vi "ATF Storage-RT_Main.vi"   [LabVIEW 2022 SP3]
uses:
  RT Controls/ATF Storage-RT main.ctl
  RT Support/ATF Storage-RT_Global_R.vi
panel:
  # "RT main ATF-Storage"
types:
  T1 = typedef "ATF Storage-RT main.ctl" = enum16{"initialise", "Wait for connection", "Wait for command"}
  T2 = enum16{"Init", "Read 'All'", "Read 'n'", "Read '1'", "Write '1'", "Write 'n'", "Write 'All'"}
  T3 = cluster{"Drive Control":cluster{"En_Drive_A":bool, "En_Drive_L":bool, "Exit_Drive_A":bool, "Exit_Drive_L":bool}, "Drive_ATF Control":cluster{"S.Freq":dbl, "Ramp up Time":dbl, "Ramp down Time":dbl, "Drive Speed":dbl, "Drive condition":dbl}, "Drive_LOX Control":cluster{"S.Freq":dbl, "Ramp up Time":dbl, "Ramp down Time":dbl, "Drive Speed":dbl, "Drive condition":dbl}, "Aconnection ID":refnum<k5>, "Lconnection ID":refnum<k5>, "Loop Control":cluster{"Start DAQ":bool, "Stop DAQ":bool, "RT Stop":bool, "RT Exit":bool, "Start Seq":bool}}
  T4 = typedef "ATF Storage-Data FIFO.ctl" = cluster{"RD":cluster{"AI_V_Data RD":refnum<queue>, "AI_C_Data RD":refnum<queue>, "AO_Data RD":refnum<queue>, "DI_Data RD":refnum<queue>, "ACC_Data RD":refnum<queue>, "TC_Data RD":refnum<queue>, "Drive_A_C RD":refnum<queue>, "Drive_A_D RD":refnum<queue>, "Drive_L_C RD":refnum<queue>, "Drive_L_D RD":refnum<queue>, "DI Data":refnum<queue>, "DO_Data RD":refnum<queue>}, "ERR":refnum<queue>}
  T5 = cluster{"Channel List":cluster{"AI Channel list":tag[], "AO Channel list":tag[], "DO Channel list ":tag[], "DI Channel list":tag[]}, "Device List":cluster{"AO Cards":tag[], "AI Cards":tag[], "DI Cards":tag[], "DO Cards":tag[]}}
  T6 = cluster{"AO config":cluster{"Channel_Name":string, "Channel_Number":string, "Default_Value":dbl, "Units":string}[], "AI config":cluster{"Channel_Name":string, "Channel_Number":string, "Pre_Scale_min":dbl, "Pre_Scale_max":dbl, "Sensor_min":dbl, "Sensor_max":dbl, "Units":string}[], "DI config":cluster{"Channel_Name":string, "Channel_Number":string, "Default_Value":bool, "DI invert?":bool}[], "DO config":cluster{"Channel_Name":string, "Channel_Number":string, "Default_Value":bool, "DO invert?":bool}[], "TC config":cluster{"Channel_Name":string, "Channel_Number":string, "Pre_Scale_min":dbl, "Pre_Scale_max":dbl, "units":i32, " type":i32}[], "ACC config":cluster{"Channel_Name":string, "Channel_Number":string, "Pre_Scale_min":dbl, "Pre_Scale_max":dbl, "Terminal configuration":i32, "Sensitivity":dbl, "Sensitivity units":i32}[], "SG config":cluster{"Channel_Name":string, "Channel_Number":string, "Pre_Scale_min":dbl, "Pre_Scale_max":dbl}[], "Strain Gauge Settings":cluster{"poisson ratio":dbl, "nominal gage resistance":dbl, "gage factor":dbl}, "Bridge Settings":cluster{"voltage excitation value":dbl, "voltage excitation source":i32, "initial bridge voltage":dbl, "lead wire resistance":dbl, "strain configuration":i32}, "Sample Rate":cluster{"AI Sample Rate":dbl[], "AO Sample Rate":dbl[], "DI Sample Rate":dbl[], "TC Sample Rate":dbl[], "DO Sample Rate":dbl[], "SG Sample Rate":dbl[], "ACC Sample Rate":dbl[]}}
  T7 = enum16{"Init", "Read", "Write 'All'", "Write 'n'", "Write Safe Value", "Write Start Time", "Overwrite Pattern", "Overwrite Pattern with Start", "Append Pattern", "Start Pattern Mode", "Abort Pattern Mode", "Read 1"}
  T8 = cluster{"Start DAQ":bool, "Stop DAQ":bool, "RT Stop":bool, "RT Exit":bool, "Start Seq":bool}
  T9 = cluster{"AO Cards":tag[], "AI Cards":tag[], "DI Cards":tag[], "DO Cards":tag[]}
  T10 = cluster{"AI Channel list":tag[], "AO Channel list":tag[], "DO Channel list ":tag[], "DI Channel list":tag[]}
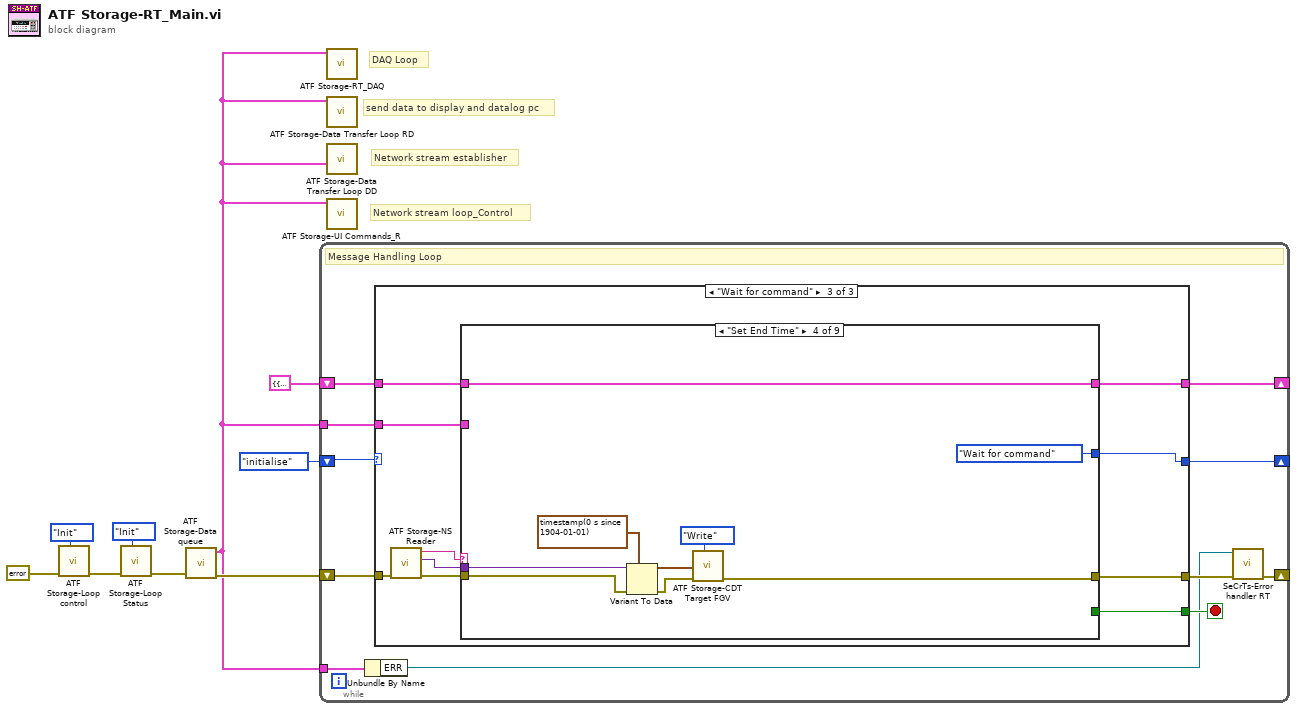
[diagram p0: block diagram]
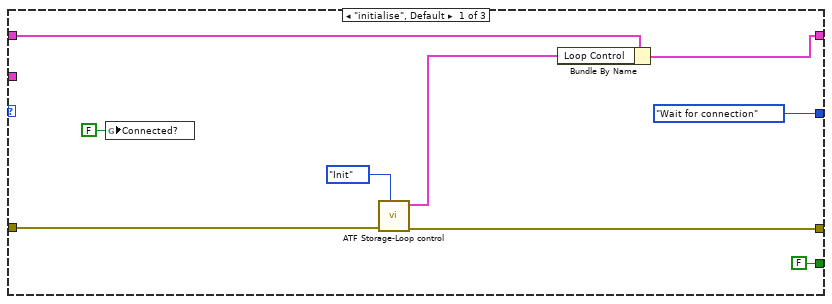
[diagram p2: hidden frame]
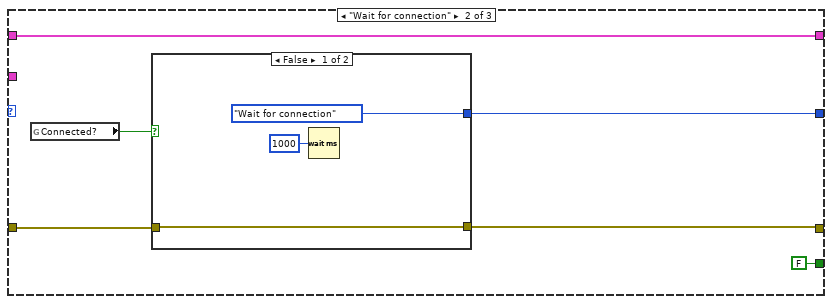
[diagram p3: hidden frame]
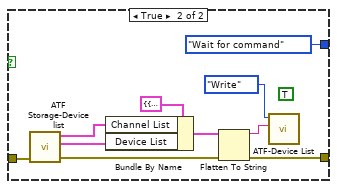
[diagram p4: hidden frame]
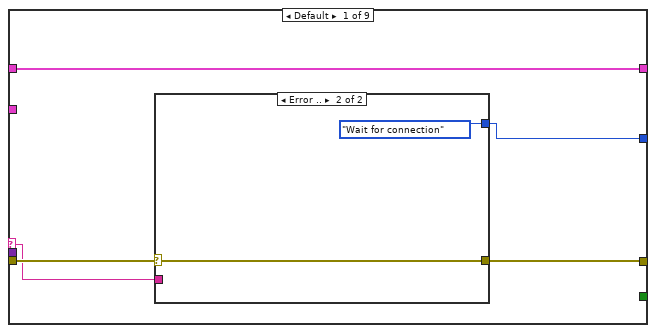
[diagram p5: hidden frame]
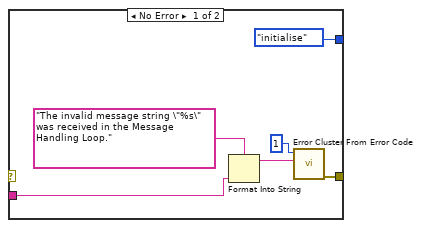
[diagram p6: hidden frame]
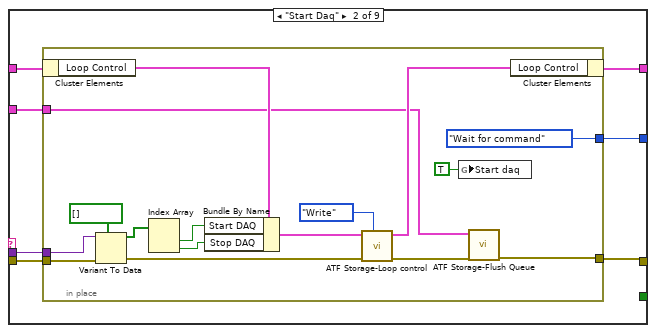
[diagram p7: hidden frame]
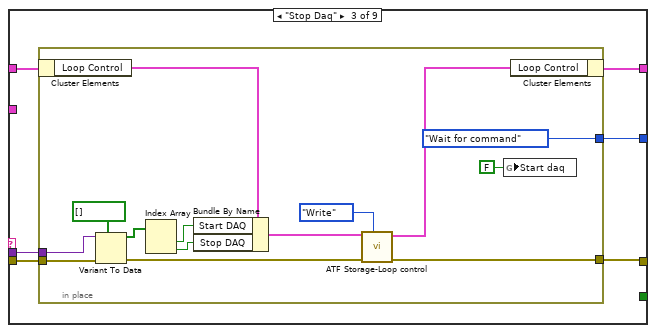
[diagram p8: hidden frame]
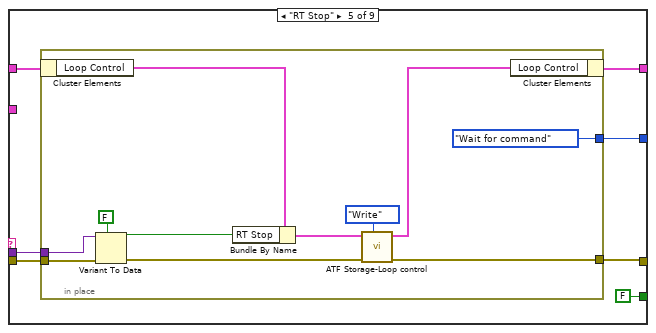
[diagram p9: hidden frame]
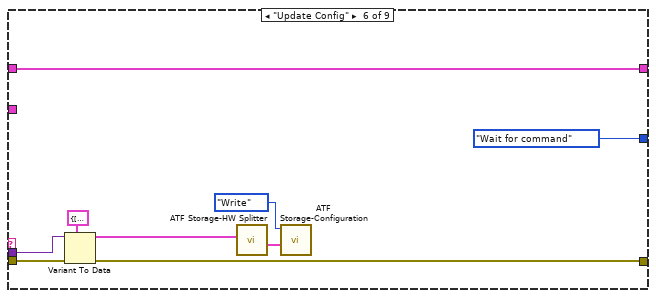
[diagram p10: hidden frame]
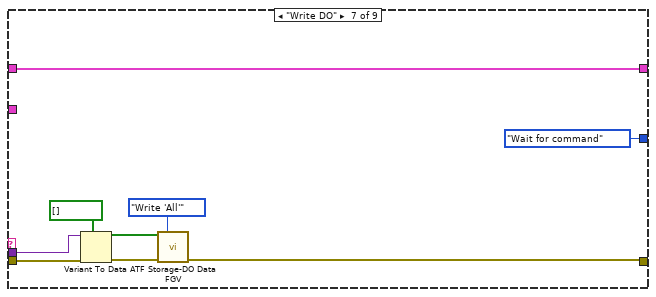
[diagram p11: hidden frame]
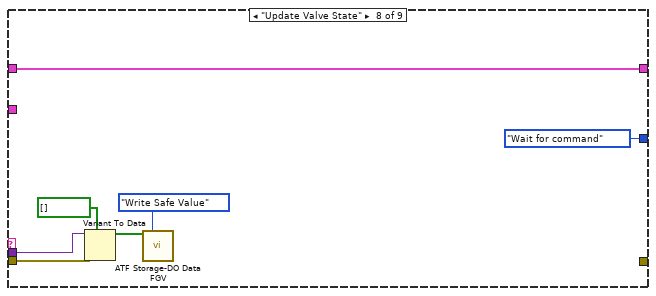
[diagram p12: hidden frame]
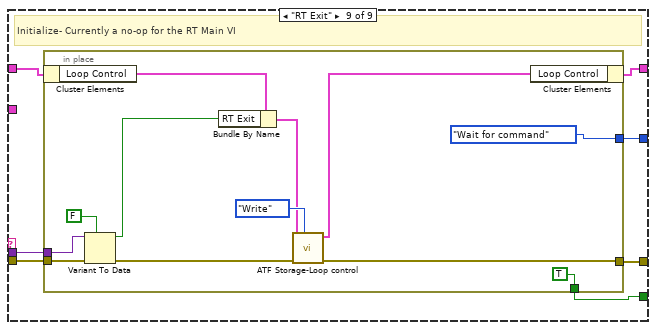
[diagram p13: hidden frame]
diagram:
  # "send data to display and datalog pc"
  # "Network stream establisher"
  # "DAQ Loop"
  # "Network stream loop_Control"
  n1 = call "ATF Storage-Loop control.vi"("Action"=enum16{"Init", "Write", "Read"}."Init", "error in (no error)"=errorcluster {"status"=FALSE, "code"=0, "source"=""} ("error constant")) -> ("error Out"=w3:errorcluster)  [unwired: 8 in, 1 out]
  n2 = call "ATF Storage-Loop Status.vi"("Option"=T2."Init", "error in (no error)"=w3) -> ("error out"=w6:errorcluster)  [unwired: 7 in, 2 out]
  n3 = call "ATF Storage-Data queue.vi"("error in"=w6) -> ("Data FIFO Ref"=w1:T4, "error out"=w8:errorcluster)  [unwired: 8 in]
  n4 = while {
    shift-right: [w15] -> _
    shift-left: w8 -> [w20]
    shift-right: [w17] -> _
    shift-left: T3 {"Drive Control"={"En_Drive_A"=FALSE, "En_Drive_L"=FALSE, "Exit_Drive_A"=FALSE, "Exit_Drive_L"=FALSE}, "Drive_ATF Control"={"S.Freq"=0.0, "Ramp up Time"=0.0, "Ramp down Time"=0.0, "Drive Speed"=0.0, "Drive condition"=0.0}, "Drive_LOX Control"={"S.Freq"=0.0, "Ramp up Time"=0.0, "Ramp down Time"=0.0, "Drive Speed"=0.0, "Drive condition"=0.0}, "Aconnection ID"=refnum, "Lconnection ID"=refnum, "Loop Control"={"Start DAQ"=FALSE, "Stop DAQ"=FALSE, "RT Stop"=FALSE, "RT Exit"=FALSE, "Start Seq"=FALSE}} -> [w18]
    tunnel: w1 -> [w14]
    shift-right: [w12] -> _
    shift-left: ATF_Storage-RT_main."initialise" -> [w13]
    tunnel: w1 -> [w11]
    stop <- w19 stop-if-true
    # "Message Handling Loop"
    n5 = Unbundle By Name(w11) -> ("ERR"=w10:refnum<queue>)
    n6 = case shown="\"Wait for command\"" w13 {
      tunnel: w20 -> [w25 w34 w53]
      tunnel: [FALSE FALSE w58] -> w19
      tunnel: w18 -> [w23 w31 w57]
      tunnel: [w22 w31 w56] -> w17
      tunnel: [w24 w33 w55] -> w16
      tunnel: w14 -> [_ _ w54]
      tunnel: [ATF_Storage-RT_main."Wait for connection" w32 w49] -> w12
      frame "initialise", Default {
        n7 = global write "ATF Storage-RT_Global_R.vi" "Connected?"(FALSE ("Connected?")) -> ()
        n8 = call "ATF Storage-Loop control.vi"("Action"=enum16{"Init", "Write", "Read"}."Init", "error in (no error)"=w25) -> ("error Out"=w24:errorcluster, "Loop Control out"=w21:T8)  [unwired: 8 in]
        n9 = Bundle By Name(cluster=w23, "Loop Control"=w21) -> (w22:T3)
      }
      frame "Wait for connection" {
        n10 = global read "ATF Storage-RT_Global_R.vi" "Connected?"() -> (w35:bool)
        n11 = case shown="False" w35 {
          tunnel: w34 -> [w38 w42]
          tunnel: [w38 w40] -> w33
          tunnel: [ATF_Storage-RT_main."Wait for connection" ATF_Storage-RT_main."Wait for command"] -> w32
          frame False {
            n12 = Wait (ms)(milliseconds to wait=u32 1000) -> ()  [unwired: 1 out]
          }
          frame True {
            (unwired) TRUE ("Connected?")
            n13 = call "ATF Storage-Device list.vi"("error in (no error)"=w42) -> ("error out"=w41:errorcluster, "Device List"=w47:T9, "Channel List"=w48:T10)  [unwired: 8 in]
            n14 = Bundle By Name(cluster=T5 {"Channel List"={"AI Channel list"=[], "AO Channel list"=[], "DO Channel list "=[], "DI Channel list"=[]}, "Device List"={"AO Cards"=[], "AI Cards"=[], "DI Cards"=[], "DO Cards"=[]}}, "Channel List"=w48, "Device List"=w47) -> (w44:T5)
            n15 = Flatten To String(anything=w44, error in (no error)=w41) -> (data string=w43:string, error out=w40:errorcluster)  [unwired: 2 in, 1 out]
            n16 = call "ATF-Device List.vi"("DL"=w43, "Enum"=enum16{"Write", "Read"}."Write") -> ()  [unwired: 8 in, 2 out]
          }
        }
      }
      frame "Wait for command" {
        n17 = call "ATF Storage-NS Reader.vi"("error in (no error)"=w53) -> ("error IO"=w52:errorcluster, "Message Data"=w51:variant, "Message"=w50:string)  [unwired: 8 in]
        n18 = case shown="\"Set End Time\"" w50 {
          selector: w50 -> [w59 _ _ _ _ _ _ _ _]
          tunnel: w51 -> [_ w76 w98 w122 w128 w147 w157 w163 w172]
          tunnel: w52 -> [w60 w78 w100 w121 w130 w148 w158 w165 w173]
          tunnel: [w61 w77 w99 w117 w129 w145 w154 _ w171] -> w55
          tunnel: [_ _ _ _ FALSE _ _ _ w170] -> w58
          tunnel: w57 -> [w63 w75 w97 w123 w127 w150 w159 w166 w169]
          tunnel: [w63 w74 w96 w123 w126 w150 w159 w166 w168] -> w56
          tunnel: w54 -> [_ w73 _ _ _ _ _ _ _]
          tunnel: [w62 w72 w95 ATF_Storage-RT_main."Wait for command" w124 ATF_Storage-RT_main."Wait for command" ATF_Storage-RT_main."Wait for command" ATF_Storage-RT_main."Wait for command" w167] -> w49
          frame Default {
            n19 = case shown="Error .." w60 {
              selector: w60 -> [_ w71]
              tunnel: w59 -> [w66 _]
              tunnel: [w65 w71] -> w61
              tunnel: [ATF_Storage-RT_main."initialise" ATF_Storage-RT_main."Wait for connection"] -> w62
              frame No Error {
                n20 = Format Into String(format string="The invalid message string \"%s\" was received in the Message Handling Loop." ("Unknown Message Error Text"), w66) -> (resulting string=w67:string)  [unwired: 2 in, 1 out]
                n21 = call <vilib>:"Error Cluster From Error Code.vi"("error message (\"\")"=w67, "error code (0)"=1) -> ("error out"=w65:errorcluster)  [unwired: 7 in]
              }
              frame Error {
              }
            }
          }
          frame "Start Daq" {
            n22 = in-place {
              in-place-border: w78 -> [w93]
              in-place-border: [w82] -> w77
              in-place-border: w76 -> [w90]
              in-place-border: w73 -> [w81]
              in-place-border: [ATF_Storage-RT_main."Wait for command"] -> w72
              n23 = in-place-cluster #1(w75) -> ("Loop Control"=w89:T8)
              n24 = Variant To Data(error in=w93, type=bool[] [], Variant=w90) -> (data=w86:bool[], error out=w91:errorcluster)
              n25 = Index Array(array=w86) -> (element #1=w85:bool, element #2=w84:bool)  [unwired: 2 in]
              n26 = Bundle By Name(cluster=w89, "Start DAQ"=w85, "Stop DAQ"=w84) -> (w88:T8)
              n27 = call "ATF Storage-Loop control.vi"("Action"=enum16{"Init", "Write", "Read"}."Write", "error in (no error)"=w91, "Loop Control In"=w88) -> ("error Out"=w83:errorcluster, "Loop Control out"=w87:T8)  [unwired: 7 in]
              n28 = global write "ATF Storage-RT_Global_R.vi" "Start daq"(TRUE ("Start daq")) -> ()
              n29 = call "ATF Storage-Flush Queue.vi"("error in (no error)"=w83, "Data FIFO Ref"=w81) -> ("error out"=w82:errorcluster)  [unwired: 9 in]
              n30 = in-place-cluster #1("Loop Control"=w87) -> (w74:T3)
            }
          }
          frame "Stop Daq" {
            n31 = in-place {
              in-place-border: w100 -> [w113]
              in-place-border: [w110] -> w99
              in-place-border: w98 -> [w109]
              in-place-border: [ATF_Storage-RT_main."Wait for command"] -> w95
              n32 = in-place-cluster #2(w97) -> ("Loop Control"=w108:T8)
              n33 = Variant To Data(error in=w113, type=bool[] [], Variant=w109) -> (data=w105:bool[], error out=w111:errorcluster)
              n34 = Index Array(array=w105) -> (element #1=w104:bool, element #2=w103:bool)  [unwired: 2 in]
              n35 = Bundle By Name(cluster=w108, "Start DAQ"=w104, "Stop DAQ"=w103) -> (w107:T8)
              n36 = call "ATF Storage-Loop control.vi"("Action"=enum16{"Init", "Write", "Read"}."Write", "error in (no error)"=w111, "Loop Control In"=w107) -> ("error Out"=w110:errorcluster, "Loop Control out"=w106:T8)  [unwired: 7 in]
              n37 = global write "ATF Storage-RT_Global_R.vi" "Start daq"(FALSE ("Start daq")) -> ()
              n38 = in-place-cluster #2("Loop Control"=w106) -> (w96:T3)
            }
          }
          frame "Set End Time" {
            n39 = Variant To Data(error in=w121, type=timestamp(0 s since 1904-01-01) ("current time"), Variant=w122) -> (data=w119:timestamp, error out=w118:errorcluster)
            n40 = call "ATF Storage-CDT Target FGV.vi"("Enum"=enum16{"Write", "Read", "Init"}."Write", "error in"=w118, "Time Stamp"=w119) -> ("error out"=w117:errorcluster)  [unwired: 7 in, 1 out]
          }
          frame "RT Stop" {
            n41 = in-place {
              in-place-border: w130 -> [w140]
              in-place-border: [w136] -> w129
              in-place-border: w128 -> [w135]
              in-place-border: [ATF_Storage-RT_main."Wait for command"] -> w124
              n42 = in-place-cluster #3(w127) -> ("Loop Control"=w134:T8)
              n43 = Variant To Data(error in=w140, type=FALSE, Variant=w135) -> (data=w139:bool, error out=w137:errorcluster)
              n44 = Bundle By Name(cluster=w134, "RT Stop"=w139) -> (w132:T8)
              n45 = call "ATF Storage-Loop control.vi"("Action"=enum16{"Init", "Write", "Read"}."Write", "error in (no error)"=w137, "Loop Control In"=w132) -> ("error Out"=w136:errorcluster, "Loop Control out"=w133:T8)  [unwired: 7 in]
              n46 = in-place-cluster #3("Loop Control"=w133) -> (w126:T3)
            }
          }
          frame "Update Config" {
            n47 = Variant To Data(error in=w148, type=T6 {"AO config"=[], "AI config"=[], "DI config"=[], "DO config"=[], "TC config"=[{"Channel_Name"="", "Channel_Number"="", "Pre_Scale_min"=0.0, "Pre_Scale_max"=0.0, "units"=4, " type"=7}], "ACC config"=[], "SG config"=[], "Strain Gauge Settings"={"poisson ratio"=0.3, "nominal gage resistance"=120.0, "gage factor"=2.08}, "Bridge Settings"={"voltage excitation value"=3.3, "voltage excitation source"=10200, "initial bridge voltage"=0.0, "lead wire resistance"=1.7, "strain configuration"=10271}, "Sample Rate"={"AI Sample Rate"=[], "AO Sample Rate"=[], "DI Sample Rate"=[], "TC Sample Rate"=[], "DO Sample Rate"=[], "SG Sample Rate"=[], "ACC Sample Rate"=[]}} ("Config in"), Variant=w147) -> (data=w144:T6, error out=w145:errorcluster)
            n48 = call "ATF Storage-HW Splitter.vi"("data"=w144) -> ("Storage HW"=w142:T6)  [unwired: 9 in, 1 out]
            n49 = call "ATF Storage-Configuration.vi"("Config in"=w142, "Enum"=enum16{"Write", "Read"}."Write") -> ()  [unwired: 9 in, 1 out]
          }
          frame "Write DO" {
            n50 = Variant To Data(error in=w158, type=bool[] [] ("DO Array"), Variant=w157) -> (data=w153:bool[], error out=w155:errorcluster)
            n51 = call "ATF Storage-DO Data FGV.vi"("DO Values In"=w153, "Option"=T7."Write 'All'", "error in (no error)"=w155) -> ("error out"=w154:errorcluster)  [unwired: 6 in, 6 out]
          }
          frame "Update Valve State" {
            n52 = Variant To Data(error in=w165, type=bool[] [], Variant=w163) -> (data=w162:bool[])  [unwired: 1 out]
            n53 = call "ATF Storage-DO Data FGV.vi"("DO Values In"=w162, "Option"=T7."Write Safe Value") -> ()  [unwired: 7 in, 7 out]
          }
          frame "RT Exit" {
            # "Initialize- Currently a no-op for the RT Main VI"
            n54 = in-place {
              in-place-border: w173 -> [w184]
              in-place-border: w172 -> [w182]
              in-place-border: [w180] -> w171
              in-place-border: [TRUE] -> w170
              in-place-border: [ATF_Storage-RT_main."Wait for command"] -> w167
              n55 = in-place-cluster #4(w169) -> ("Loop Control"=w177:T8)
              n56 = Variant To Data(error in=w184, type=FALSE, Variant=w182) -> (data=w181:bool, error out=w183:errorcluster)
              n57 = Bundle By Name(cluster=w177, "RT Exit"=w181) -> (w176:T8)
              n58 = call "ATF Storage-Loop control.vi"("Action"=enum16{"Init", "Write", "Read"}."Write", "error in (no error)"=w183, "Loop Control In"=w176) -> ("error Out"=w180:errorcluster, "Loop Control out"=w175:T8)  [unwired: 7 in]
              n59 = in-place-cluster #4("Loop Control"=w175) -> (w168:T3)
            }
          }
        }
      }
    }
    n60 = call "SeCrTs-Error handler RT.vi"("error in"=w16, "Message Queue"=w10) -> ("error out"=w15:errorcluster)  [unwired: 8 in, 1 out]
  }
  n61 = call "ATF Storage-RT_DAQ.vi"("Data FIFO Ref"=w1) -> ()  [unwired: 10 in, 1 out]
  n62 = call "ATF Storage-Data Transfer Loop RD.vi"("Data FIFO Ref"=w1) -> ()  [unwired: 11 in]
  n63 = call "ATF Storage-Data Transfer Loop DD.vi"("Data FIFO Ref"=w1) -> ()  [unwired: 11 in]
  n64 = call "ATF Storage-UI Commands_R.vi"("Data FIFO Ref"=w1) -> ()  [unwired: 11 in]
